vi "string_split.vi"(1 "input":string) -> (0 "output":string[](array[string]))   [LabVIEW 2012]
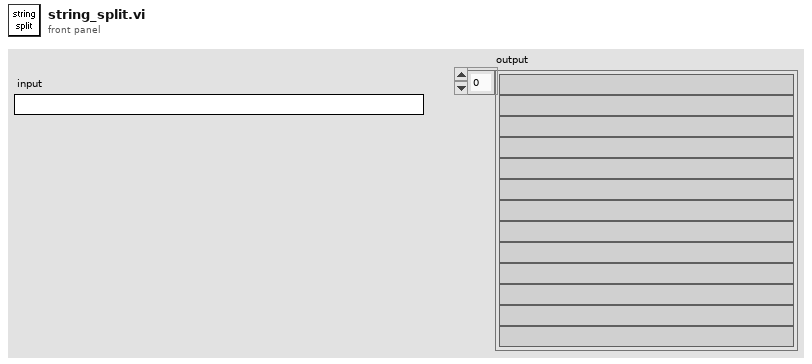
[diagram p1: front panel]
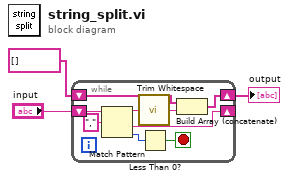
[diagram p0: block diagram]
diagram:
  n1 = while {
    shift-right: [w9] -> _
    shift-left: "input" -> [w8]
    shift-right: [w7] -> w2
    shift-left: string[] [] -> [w6]
    stop <- w10 stop-if-true
    n2 = Match Pattern(string=w8, regular expression=",") -> (before substring=w5:string, after substring=w9:string, offset past match=w11:i32)  [unwired: 1 in, 1 out]
    n3 = call <vilib>:"Trim Whitespace.vi"("string"=w5) -> ("trimmed string"=w4:string)  [unwired: 1 in]
    n4 = Less Than 0?(x=w11) -> (x < 0?=w10:bool)
    n5 = Build Array (concatenate)(w6, w4) -> (w7:string[])
  }
  "output" <- w2
